vi "App Status Globals.vi"(0 "App Status Actions":T5=enum."Get Status", 1 "LBCB Number":T4, 5 "Status\nSetting":bool, 7 "App State":T2=enum."Initializing Displays", 9 "App Status In":T1={"Running"=TRUE, "Controlling L2"=FALSE, "Autobalance L2"=FALSE, "Data Acquisition"=FALSE, " App State"=enum."Initializing Displays", "DAQ Started"=FALSE, "LBCB 1 State"=enum."Idle", "LBCB 2 State"=enum."Idle", "Controlling L1"=FALSE, "Autobalance L1"=FALSE, "Cartesian Type"=FALSE, "Continuous Logging"=FALSE, "Step Logging"=FALSE, "Voltage Logging"=FALSE, "Mixed Mode Logging"=FALSE, "DAQ Link"=FALSE, "NTCP Link "=FALSE}, 11 "error in (no error)":errorcluster, 12 "LBCB State":T3) -> (4 "App Status Out":T1={"Running"=TRUE, "Controlling L2"=FALSE, "Autobalance L2"=FALSE, "Data Acquisition"=FALSE, " App State"=enum."Initializing Displays", "DAQ Started"=FALSE, "LBCB 1 State"=enum."Idle", "LBCB 2 State"=enum."Idle", "Controlling L1"=FALSE, "Autobalance L1"=FALSE, "Cartesian Type"=FALSE, "Continuous Logging"=FALSE, "Step Logging"=FALSE, "Voltage Logging"=FALSE, "Mixed Mode Logging"=FALSE, "DAQ Link"=FALSE, "NTCP Link "=FALSE}, 15 "error out":errorcluster)   [LabVIEW 2009]
uses:
  App Status.ctl
  AppStates.ctl
  Lbcb Control Loop States.ctl
  App Status Actions.ctl
  Data Access Objects/Metadata/LBCB Number.ctl
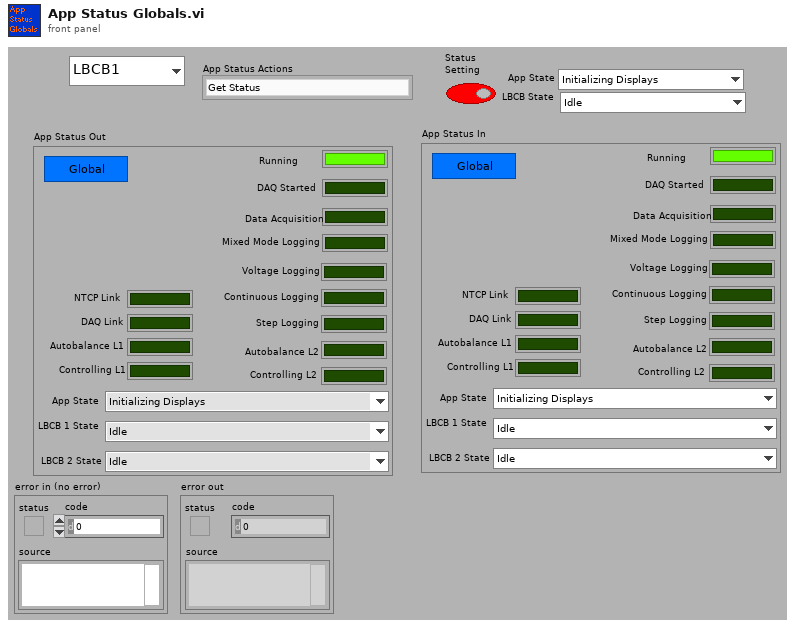
[diagram p1: front panel]
types:
  T1 = typedef "App Status.ctl" = cluster{"Running":bool, "Controlling L2":bool, "Autobalance L2":bool, "Data Acquisition":bool, " App State":T2, "DAQ Started":bool, "LBCB 1 State":T3, "LBCB 2 State":T3, "Controlling L1":bool, "Autobalance L1":bool, "Cartesian Type":bool, "Continuous Logging":bool, "Step Logging":bool, "Voltage Logging":bool, "Mixed Mode Logging":bool, "DAQ Link":bool, "NTCP Link ":bool}
  T2 = typedef "AppStates.ctl" = enum16{"Starting OM", "Initializing Displays", "Setting up Archiving", "Setting Up DAQ Channels", "Start DAQ", "DAQ Starting", "Controlling LBCBs", "Stopping OM"}
  T3 = typedef "Lbcb Control Loop States.ctl" = enum16{"Idle", "Start Selected", "Load Last Command", "Start Autobalancing", "Autobalancing", "Control Loop Initialized", "Control Enabled"}
  T4 = typedef "LBCB Number.ctl" = enum16{"LBCB1", "LBCB2"}
  T5 = typedef "App Status Actions.ctl" = enum16{"Init", "Get Status", "Running", "Control", "Autobalanced", "Data Acquisition", "Set App State", "DAQ Started", "Set LBCB State", "Set All", "Set Cont Logging", "Set Step Logging", "Set MM Logging", "Set Volt Logging", "Set Cart Type", "Set DAQ Link", "Set NTCP Link"}
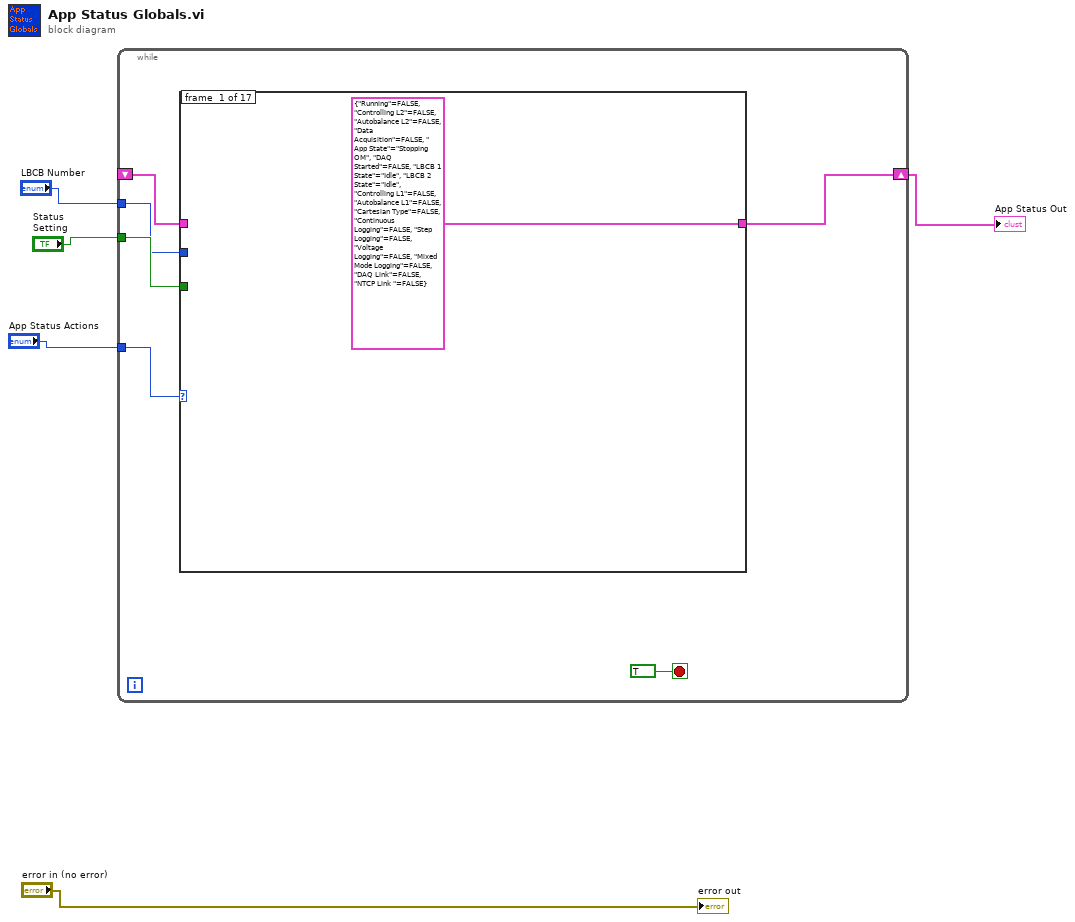
[diagram p0: block diagram]
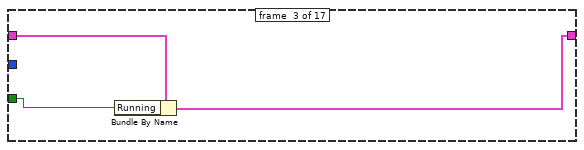
[diagram p3: hidden frame]
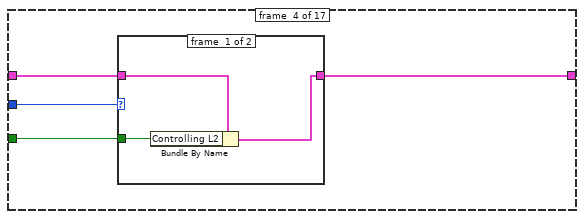
[diagram p4: hidden frame]
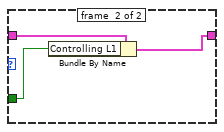
[diagram p5: hidden frame]
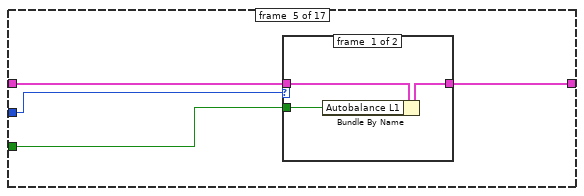
[diagram p6: hidden frame]
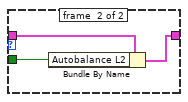
[diagram p7: hidden frame]
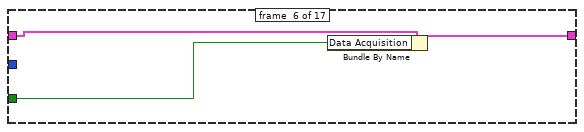
[diagram p8: hidden frame]
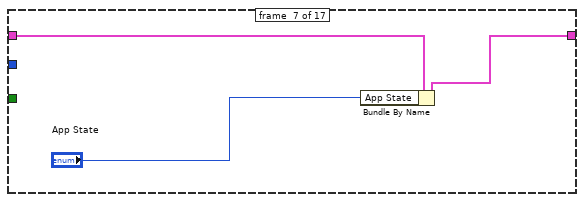
[diagram p9: hidden frame]
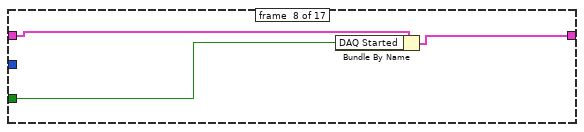
[diagram p10: hidden frame]
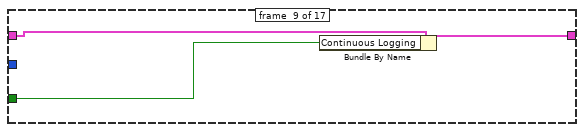
[diagram p11: hidden frame]
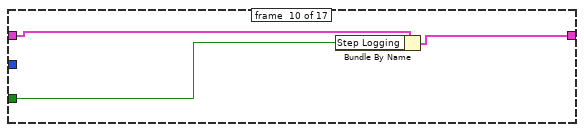
[diagram p12: hidden frame]
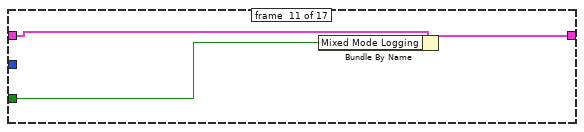
[diagram p13: hidden frame]
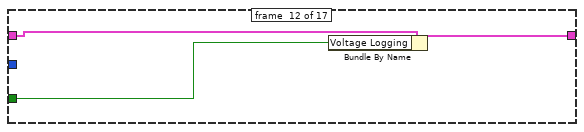
[diagram p14: hidden frame]
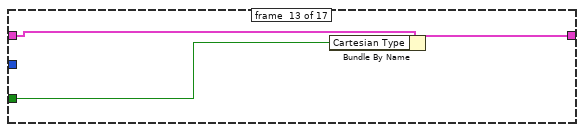
[diagram p15: hidden frame]
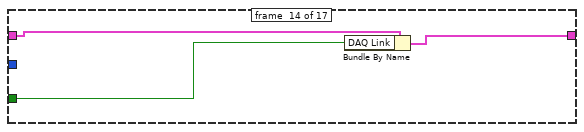
[diagram p16: hidden frame]
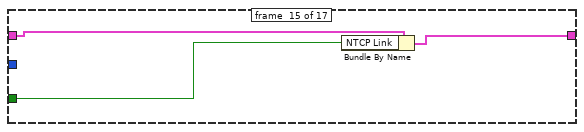
[diagram p17: hidden frame]
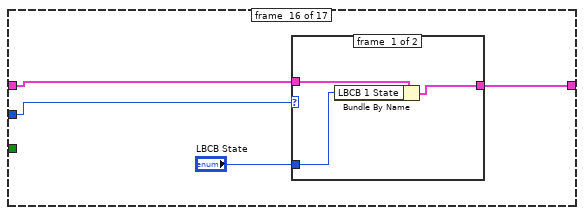
[diagram p18: hidden frame]
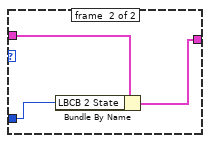
[diagram p19: hidden frame]
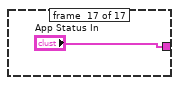
[diagram p20: hidden frame]
diagram:
  n1 = while {
    tunnel: "App Status Actions" -> [w10]
    tunnel: "Status\nSetting" -> [w9]
    shift-right: [w6] -> w1
    shift-left: _ -> [w7]
    tunnel: "LBCB Number" -> [w8]
    stop <- TRUE stop-if-true
    n2 = case shown="\"Set Cart Type\"" w10 {
      tunnel: w9 -> [_ _ w16 w20 w30 w39 _ w45 w48 w51 w54 w57 w60 w63 w66 _ _]
      tunnel: [T1 {"Running"=FALSE, "Controlling L2"=FALSE, "Autobalance L2"=FALSE, "Data Acquisition"=FALSE, " App State"=enum."Stopping OM", "DAQ Started"=FALSE, "LBCB 1 State"=enum."Idle", "LBCB 2 State"=enum."Idle", "Controlling L1"=FALSE, "Autobalance L1"=FALSE, "Cartesian Type"=FALSE, "Continuous Logging"=FALSE, "Step Logging"=FALSE, "Voltage Logging"=FALSE, "Mixed Mode Logging"=FALSE, "DAQ Link"=FALSE, "NTCP Link "=FALSE} ("App Status") w13 w15 w17 w28 w37 w40 w43 w46 w49 w52 w55 w58 w61 w64 w69 "App Status In"] -> w6
      tunnel: w8 -> [_ _ _ w19 w27 _ _ _ _ _ _ _ _ _ _ w68 _]
      tunnel: w7 -> [_ w13 w14 w18 w29 w38 w41 w44 w47 w50 w53 w56 w59 w62 w65 w70 _]
      frame #0 {
      }
      frame #1 {
      }
      frame #2 {
        n3 = Bundle By Name(cluster=w14, "Running"=w16) -> (w15:T1)
      }
      frame #3 {
        n4 = case shown="\"LBCB2\"" w19 {
          tunnel: w20 -> [w23 w26]
          tunnel: w18 -> [w22 w25]
          tunnel: [w21 w24] -> w17
          frame #0 {
            n5 = Bundle By Name(cluster=w22, "Controlling L2"=w23) -> (w21:T1)
          }
          frame #1 {
            n6 = Bundle By Name(cluster=w25, "Controlling L1"=w26) -> (w24:T1)
          }
        }
      }
      frame #4 {
        n7 = case shown="\"LBCB1\"" w27 {
          tunnel: w30 -> [w33 w36]
          tunnel: w29 -> [w32 w35]
          tunnel: [w31 w34] -> w28
          frame #0 {
            n8 = Bundle By Name(cluster=w32, "Autobalance L1"=w33) -> (w31:T1)
          }
          frame #1 {
            n9 = Bundle By Name(cluster=w35, "Autobalance L2"=w36) -> (w34:T1)
          }
        }
      }
      frame #5 {
        n10 = Bundle By Name(cluster=w38, "Data Acquisition"=w39) -> (w37:T1)
      }
      frame #6 {
        n11 = Bundle By Name(cluster=w41, "App State"="App State") -> (w40:T1)
      }
      frame #7 {
        n12 = Bundle By Name(cluster=w44, "DAQ Started"=w45) -> (w43:T1)
      }
      frame #8 {
        n13 = Bundle By Name(cluster=w47, "Continuous Logging"=w48) -> (w46:T1)
      }
      frame #9 {
        n14 = Bundle By Name(cluster=w50, "Step Logging"=w51) -> (w49:T1)
      }
      frame #10 {
        n15 = Bundle By Name(cluster=w53, "Mixed Mode Logging"=w54) -> (w52:T1)
      }
      frame #11 {
        n16 = Bundle By Name(cluster=w56, "Voltage Logging"=w57) -> (w55:T1)
      }
      frame #12 {
        n17 = Bundle By Name(cluster=w59, "Cartesian Type"=w60) -> (w58:T1)
      }
      frame #13 {
        n18 = Bundle By Name(cluster=w62, "DAQ Link"=w63) -> (w61:T1)
      }
      frame #14 {
        n19 = Bundle By Name(cluster=w65, "NTCP Link"=w66) -> (w64:T1)
      }
      frame #15 {
        n20 = case shown="\"LBCB2\"" w68 {
          tunnel: w70 -> [w73 w76]
          tunnel: [w72 w75] -> w69
          tunnel: "LBCB State" -> [w71 w74]
          frame #0 {
            n21 = Bundle By Name(cluster=w73, "LBCB 1 State"=w71) -> (w72:T1)
          }
          frame #1 {
            n22 = Bundle By Name(cluster=w76, "LBCB 2 State"=w74) -> (w75:T1)
          }
        }
      }
      frame #16 {
      }
    }
  }
  "App Status Out" <- w1
  "error out" <- "error in (no error)"
